vi "GetCameraSettings.vi"(0 "Session In":T3, 5 "Array":i32[](array[numeric]), 7 "Brightness":i64(slide) scale=0.0..255.0, 9 "Contrast":dbl(slide) scale=0.0..1.0) -> (2 "Contrast":dbl, 3 "Brightness":i64, 4 "Session Out":T3, 6 "Histogram Graph":cluster{dbl[], dbl[]}(graph), 8 "Image":T4(plugin-control), 13 "Histogram Statistics":T2, 14 "Quality Check Variables":T1, 15 "error out":errorcluster)   [LabVIEW 2017]
uses:
  <vilib>/userdefined/High Color/IMAQdx.ctl
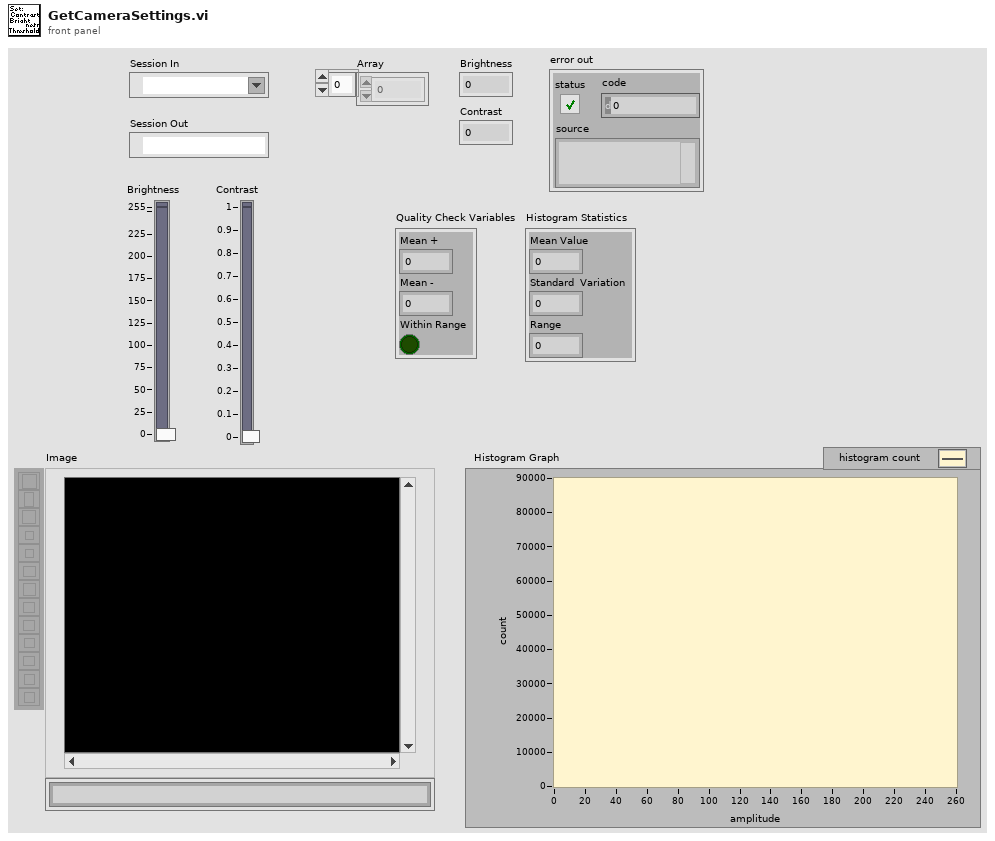
[diagram p1: front panel]
types:
  T1 = cluster{"Mean +":dbl, "Mean -":dbl, "Within Range":bool}
  T2 = cluster{"Mean Value":sgl, "Standard  Variation":sgl, "Range":sgl}
  T3 = typedef "IMAQdx.ctl" = refnum<k21>
  T4 = typedef "IMAQ Image.ctl" = refnum<image>
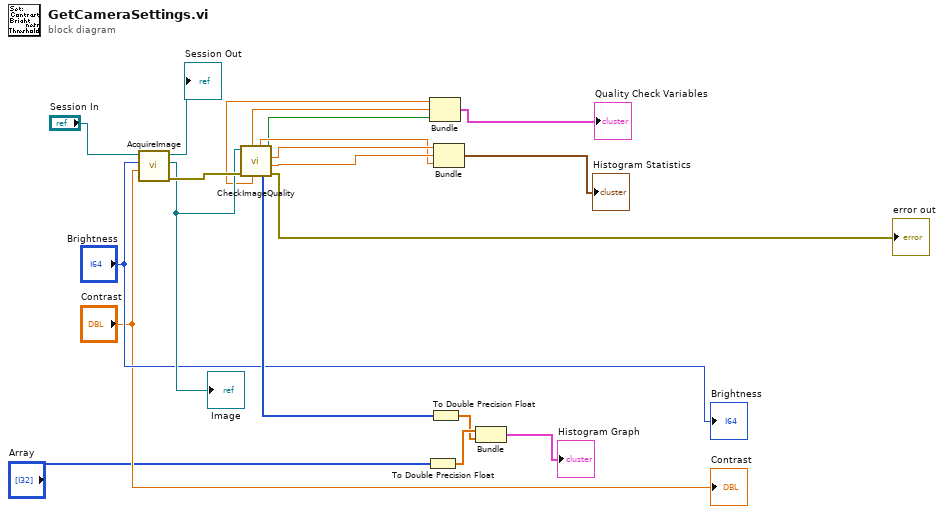
[diagram p0: block diagram]
diagram:
  n1 = call "AcquireImage.vi"("Contrast"="Contrast", "Brightness"="Brightness", "Session In"="Session In") -> ("error out"=w20:errorcluster, "Image"=w14:T4, "Session Out"=→"Session Out":T3)  [unwired: 5 in]
  "Image" <- w14
  n2 = call "CheckImageQuality.vi"("error in (no error)"=w20, "Image"=w14) -> ("error out"=→"error out":errorcluster, "Standard  Variation"=w7:sgl, "Mean Value"=w8:sgl, "Within Range"=w2:bool, "histogram"=w19:u32[], "Range"=w6:sgl, "Mean +"=w4:dbl, "Mean -"=w3:dbl)  [unwired: 2 in]
  n3 = To Double Precision Float(number="Array") -> (double precision float=w16:dbl[])
  n4 = Bundle("Mean +"=w4, "Mean -"=w3, "Within Range"=w2) -> (→"Quality Check Variables":T1)  [unwired: 1 in]
  n5 = To Double Precision Float(number=w19) -> (double precision float=w15:dbl[])
  n6 = Bundle("Mean Value"=w8, "Standard  Variation"=w7, "Range"=w6) -> (→"Histogram Statistics":T2)  [unwired: 1 in]
  n7 = Bundle(w16, w15) -> (→"Histogram Graph":cluster{dbl[], dbl[]})  [unwired: 1 in]
  "Brightness" <- "Brightness"
  "Contrast" <- "Contrast"
